vi "Test wiimote.vi"() -> ()   [LabVIEW 2010]
panel:
  out "1D Experiment":cluster{dbl[], dbl[]}[](graph)
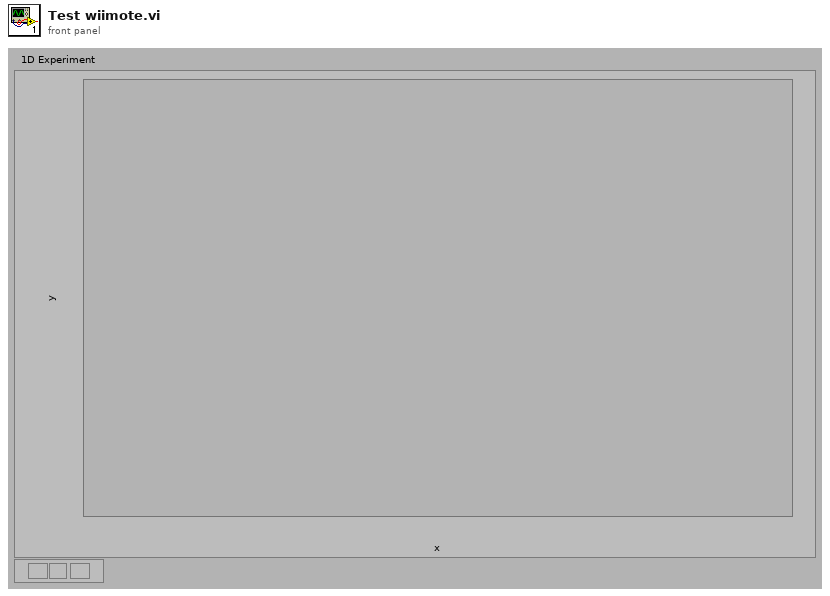
[diagram p1: front panel]
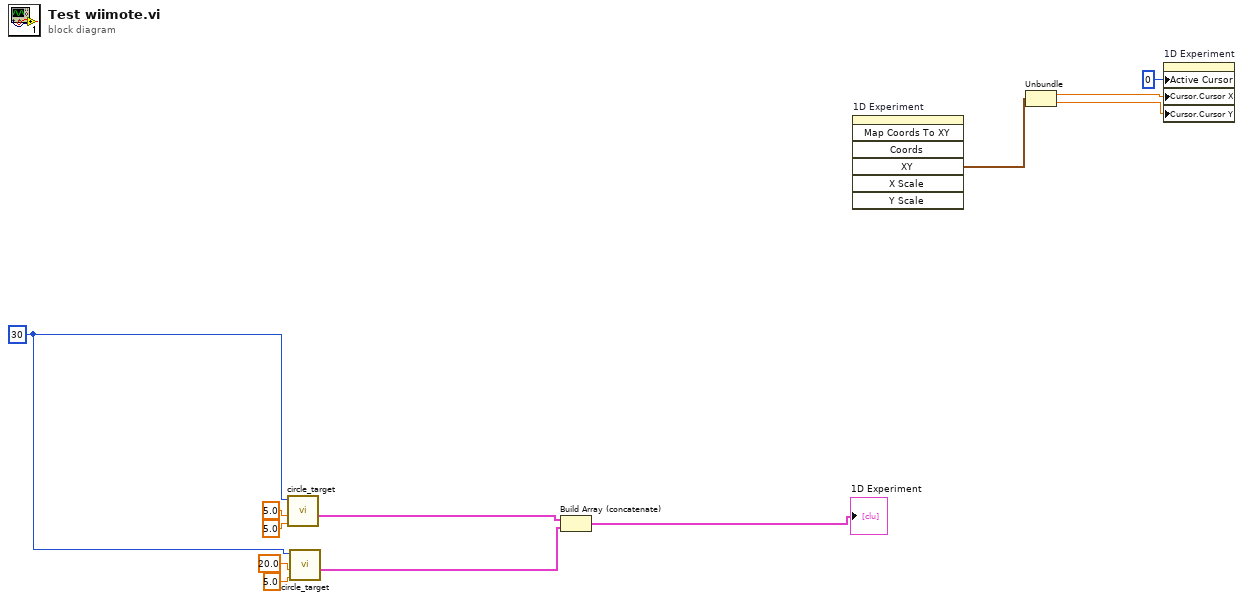
[diagram p0: block diagram]
diagram:
  w8 = 30
  n1 = call "circle_target.vi"("y0"=5.0, "x0"=5.0, "Target's width"=w8) -> ("Target plots"=w5:cluster{dbl[], dbl[]}[])  [unwired: 7 in, 1 out]
  n2 = call "circle_target.vi"("y0"=5.0, "x0"=20.0, "Target's width"=w8) -> ("Target plots"=w6:cluster{dbl[], dbl[]}[])  [unwired: 7 in, 1 out]
  n3 = Build Array (concatenate)(w5, w6) -> (→"1D Experiment":cluster{dbl[], dbl[]}[])
  n4 = invoke on="1D Experiment" class="XYGraph (strict)" method="Map Coords To XY"() -> ("XY"=w3:cluster{"X":dbl, "Y":dbl})  [unwired: 7 in, 6 out]
  n5 = Unbundle(w3) -> ("X"=w2:dbl, "Y"=w1:dbl)
  n6 = property on="1D Experiment" class="XYGraph (strict)"("Active Cursor"=u32 0, "Cursor.Cursor X"=w2, "Cursor.Cursor Y"=w1) -> ()  [unwired: 2 in, 2 out]
